vi "PH_GUI.set cluster GUI object element.vi"(1 "Ctl Refnum":refnum<vi>, 3 "Value":variant, 4 "Blinking? (false)":bool, 5 "error in":errorcluster, 7 "Grayed out? (false)":bool) -> (19 "error out":errorcluster)   [LabVIEW 2014, in "PH_Common.lvlib"]
doc: "Sets value and more for the referenced GUI object."
uses:
  PH_Common.lvlib
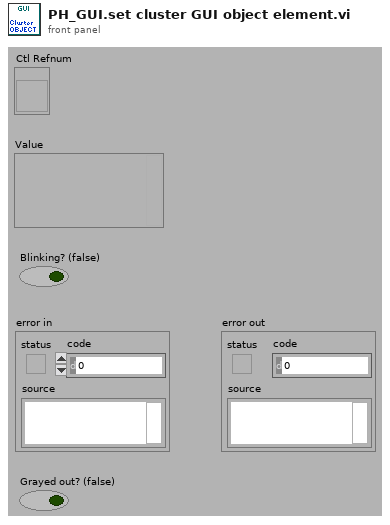
[diagram p1: front panel]
types:
  T1 = enum8{"Enabled", "Disabled", "Disabled and Grayed Out"}
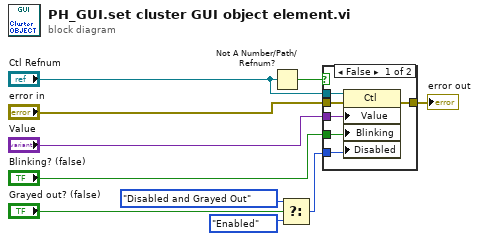
[diagram p0: block diagram]
diagram:
  n1 = Not A Number/Path/Refnum?(number/path/refnum="Ctl Refnum") -> (NaN/Path/Refnum?=w7:bool)
  n2 = Select(t=T1."Disabled and Grayed Out" ("Disabled"), s="Grayed out? (false)", f=T1."Enabled" ("Disabled")) -> (s? t:f=w10:T1)
  n3 = case shown="False" w7 {
    tunnel: "Ctl Refnum" -> [w16 _]
    tunnel: "error in" -> [w15 w17]
    tunnel: [w14 w17] -> w3
    tunnel: "Blinking? (false)" -> [w13 _]
    tunnel: "Value" -> [w12 _]
    tunnel: w10 -> [w11 _]
    frame False {
      n4 = property class="Ctl"(reference=w16, error in=w15, "Value"=w12, "Blinking"=w13, "Disabled"=w11) -> (error out=w14:errorcluster)  [unwired: 1 out]
    }
    frame True {
    }
  }
  "error out" <- w3
